vi "ATF-Combined Device List.vi"(10 "Storage":T2, 11 "Pump":T1) -> (2 "Combined Device list":T2)   [LabVIEW 2022 SP3]
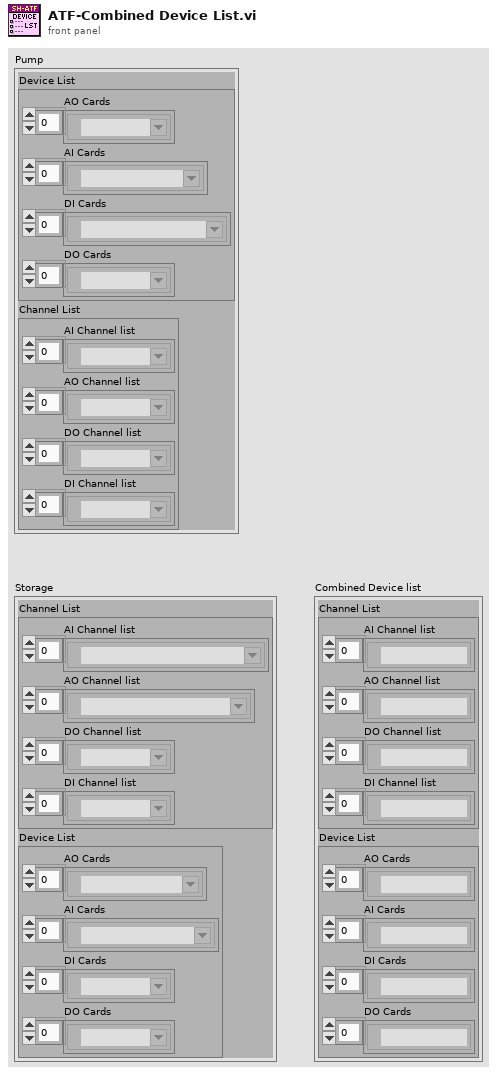
[diagram p1: front panel]
types:
  T1 = cluster{"Device List":cluster{"AO Cards":tag[], "AI Cards":tag[], "DI Cards":tag[], "DO Cards":tag[]}, "Channel List":cluster{"AI Channel list":tag[], "AO Channel list":tag[], "DO Channel list ":tag[], "DI Channel list":tag[]}}
  T2 = cluster{"Channel List":cluster{"AI Channel list":tag[], "AO Channel list":tag[], "DO Channel list ":tag[], "DI Channel list":tag[]}, "Device List":cluster{"AO Cards":tag[], "AI Cards":tag[], "DI Cards":tag[], "DO Cards":tag[]}}
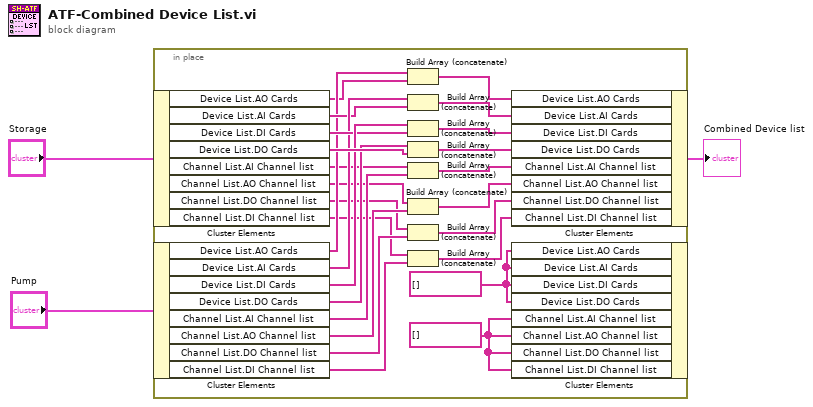
[diagram p0: block diagram]
diagram:
  n1 = in-place {
    w4 = tag[] [] ("Channel List.AI Channel list")
    w17 = tag[] [] ("Device List.AO Cards")
    n2 = in-place-cluster #1("Storage") -> ("Device List.AO Cards"=w19:tag[], "Device List.AI Cards"=w21:tag[], "Device List.DI Cards"=w25:tag[], "Device List.DO Cards"=w29:tag[], "Channel List.AI Channel list"=w15:tag[], "Channel List.AO Channel list"=w12:tag[], "Channel List.DO Channel list"=w10:tag[], "Channel List.DI Channel list"=w6:tag[])
    n3 = in-place-cluster #2("Pump") -> ("Device List.AO Cards"=w20:tag[], "Device List.AI Cards"=w23:tag[], "Device List.DI Cards"=w26:tag[], "Device List.DO Cards"=w28:tag[], "Channel List.AI Channel list"=w16:tag[], "Channel List.AO Channel list"=w11:tag[], "Channel List.DO Channel list"=w9:tag[], "Channel List.DI Channel list"=w5:tag[])
    n4 = Build Array (concatenate)(w20, w19) -> (w18:tag[])
    n5 = Build Array (concatenate)(w23, w21) -> (w22:tag[])
    n6 = Build Array (concatenate)(w26, w25) -> (w24:tag[])
    n7 = Build Array (concatenate)(w28, w29) -> (w27:tag[])
    n8 = Build Array (concatenate)(w15, w16) -> (w14:tag[])
    n9 = Build Array (concatenate)(w12, w11) -> (w13:tag[])
    n10 = Build Array (concatenate)(w10, w9) -> (w8:tag[])
    n11 = Build Array (concatenate)(w6, w5) -> (w7:tag[])
    n12 = in-place-cluster #1("Device List.AO Cards"=w18, "Device List.AI Cards"=w22, "Device List.DI Cards"=w24, "Device List.DO Cards"=w27, "Channel List.AI Channel list"=w14, "Channel List.AO Channel list"=w13, "Channel List.DO Channel list"=w8, "Channel List.DI Channel list"=w7) -> (→"Combined Device list":T2)
    n13 = in-place-cluster #2("Device List.AO Cards"=w17, "Device List.AI Cards"=w17, "Device List.DI Cards"=w17, "Device List.DO Cards"=w17, "Channel List.AI Channel list"=w4, "Channel List.AO Channel list"=w4, "Channel List.DO Channel list"=w4, "Channel List.DI Channel list"=w4) -> ()  [unwired: 1 out]
  }
